vi "K_degCtoV.vi"(3 "Temperature (degC)":dbl) -> (0 "error":i32, 1 "Voltage (mV)":sgl)   [LabVIEW 2023]
uses:
  <vilib>/Analysis/NI_AALPro.lvlib
  <vilib>/Analysis/polynomials.llb/Scalar Polynomial Evaluation (DBL).vi
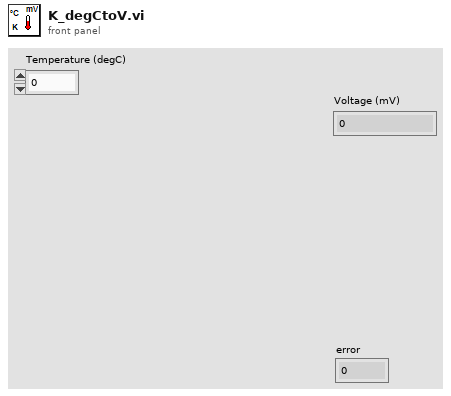
[diagram p1: front panel]
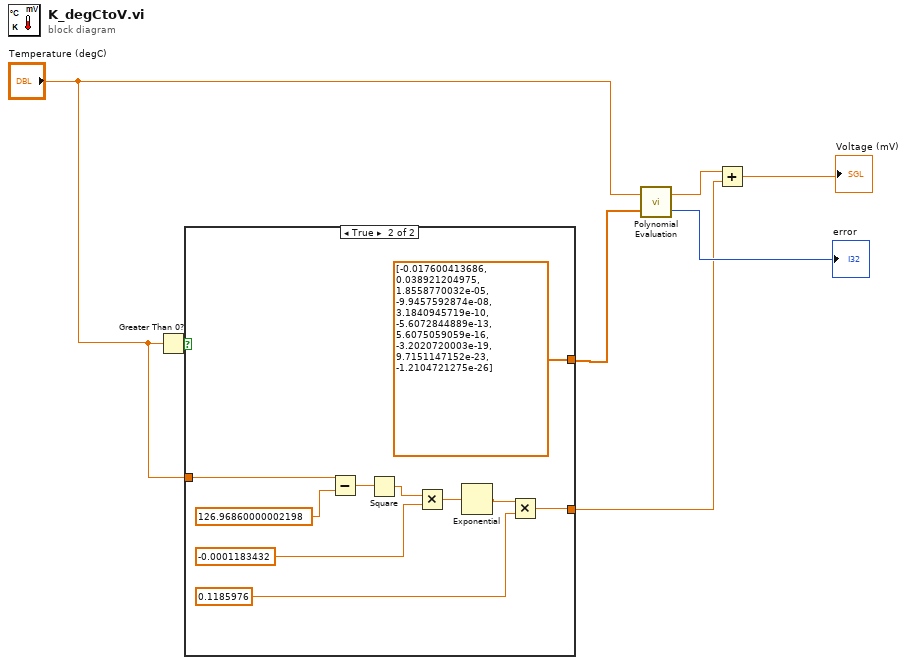
[diagram p0: block diagram]
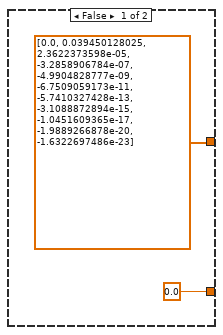
[diagram p2: hidden frame]
diagram:
  n1 = Greater Than 0?(x="Temperature (degC)") -> (x > 0?=w1:bool)
  n2 = case shown="True" w1 {
    tunnel: [dbl[] [0.0, 0.039450128025, 2.3622373598e-05, -3.2858906784e-07, -4.9904828777e-09, -6.7509059173e-11, -5.7410327428e-13, -3.1088872894e-15, -1.0451609365e-17, -1.9889266878e-20, -1.6322697486e-23] ("Coefficinets") dbl[] [-0.017600413686, 0.038921204975, 1.8558770032e-05, -9.9457592874e-08, 3.1840945719e-10, -5.6072844889e-13, 5.6075059059e-16, -3.2020720003e-19, 9.7151147152e-23, -1.2104721275e-26] ("Coefficinets")] -> w7
    tunnel: [0.0 w11] -> w2
    tunnel: "Temperature (degC)" -> [_ w18]
    frame False {
    }
    frame True {
      n3 = Subtract(x=w18, y=126.96860000002198) -> (x-y=w16:dbl)
      n4 = Square(x=w16) -> (x^2=w15:dbl)
      n5 = Multiply(x=w15, y=-0.0001183432) -> (x*y=w13:dbl)
      n6 = Exponential(1:w13) -> (0:w12:dbl)
      n7 = Multiply(x=w12, y=0.1185976) -> (x*y=w11:dbl)
    }
  }
  n8 = call-poly <vilib>:"Polynomial Evaluation.vi"("P(x)"=w7, "a"="Temperature (degC)") -> ("error"=→"error":i32, "P(a)"=w6:dbl)
  n9 = Add(x=w6, y=w2) -> (x+y=→"Voltage (mV)":dbl)
